vi "Initiate Updates.vi"(8 "error in (no error)":errorcluster, 11 "IViewable In":refnum<class "IViewable.lvclass">) -> (0 "error out":errorcluster, 3 "IViewable Out":refnum<class "IViewable.lvclass">)   [LabVIEW 2017, in "IViewable.lvlib" / "IViewable.lvclass"]
doc: "<License>\nCopyright © 2017 Composed Systems, LLC | All rights reserved\nwww.composed.io\n\nAuthor: Ethan Stern <ethan.stern@composed.io>\n\nThis software is provided \"AS IS\" WITHOUT WARRANTIES, either express or implied, AND IS FOR EDUCATIONAL PURPOSES ONLY.\n</License>"
uses:
  IViewable.lvclass
  IViewable.lvclass/IViewable.ctl
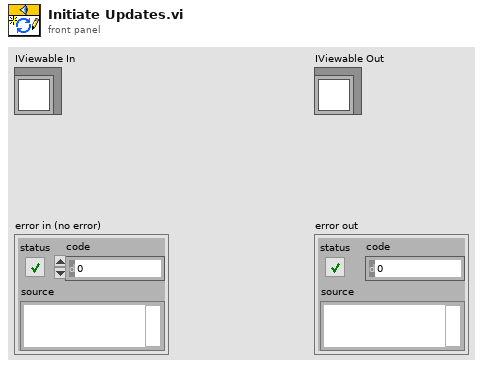
[diagram p1: front panel]
types:
  T1 = enum32{"Invalid", "Standard", "Closed", "Hidden", "Minimized", "Maximized"}
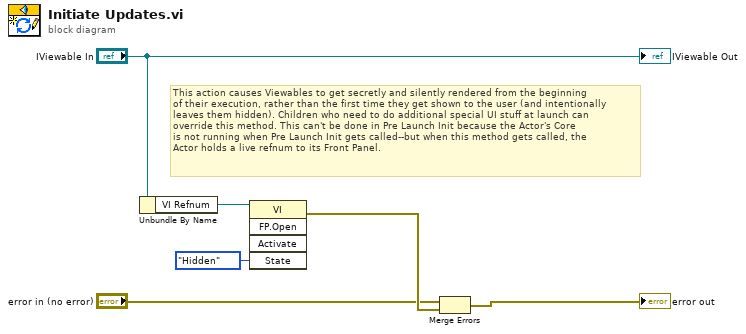
[diagram p0: block diagram]
diagram:
  # "This action causes Viewables to get secretly and silently rendered from the beginning\nof their execution, rather than the first time they get shown to the user (and intentionally\nleaves them hidden). Children who need to do additional special UI stuff at launch can\noverride this method. This can't be done in Pre Launch Init because the Actor's Core\nis not running when Pre Launch Init gets called--but when this method gets called, the\nActor holds a live refnum to its Front Panel."
  n1 = Unbundle By Name("IViewable In") -> ("VI Refnum"=w1:refnum<vi>)
  n2 = invoke class="VI" method="FP.Open"(reference=w1, "State"=T1."Hidden") -> (error out=w6:errorcluster)  [unwired: 3 in, 4 out]
  n3 = Merge Errors("error in (no error)", w6) -> (→"error out":errorcluster)
  "IViewable Out" <- "IViewable In"
